vi "DMAC U8 to DMAC U64.vi"(5 "DestinationMACAddress":u8[](array[numeric])=[3, 0, 94, 160, 3, 233] format="%02x") -> (2 "DMAC U64":u64 format="%012x")   [LabVIEW 2021, in "Networking_CIF_U.lvlib"]
uses:
  Networking_CIF_U.lvlib
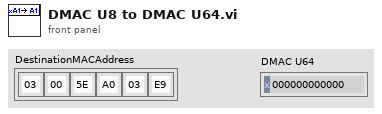
[diagram p1: front panel]
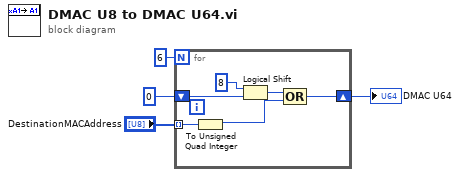
[diagram p0: block diagram]
diagram:
  n1 = for {
    N: 6 -> [_]
    tunnel: "DestinationMACAddress" -> [w10] mode=indexing
    shift-right: [w5] -> w2
    shift-left: u64 0 -> [w7]
    n2 = To Unsigned Quad Integer(1:w10) -> (0:w9:u64)
    n3 = Logical Shift(y=i16 8, x=w7) -> (x << y=w6:u64)
    n4 = Compound Arithmetic op=OR(w6, w9) -> (w5:u64)
  }
  "DMAC U64" <- w2
